vi "PBKDF2.vi"() -> ()   [LabVIEW 2013]
doc: "Implements password-based key derivation functionality, PBKDF2, by using a pseudo-random number generator based on HMACSHA1.\n\nLabVIEW implementation of the C# code example from Microsft's web site @ http://msdn.microsoft.com/en-us/library/system.security.cryptography.rfc2898derivebytes(v=VS.80).aspx\n\n1/17/2011 P. Brooks Originated."
panel:
  out "Decrypted String":string
  in  "MyIterations":i32=1000
  out "encrypted string":string
  in  "Data":string="using System;\nusing System.IO;\nusing System.Text;\nusing System.Security.Cryptography;\n\npublic class rfc2898test\n{\n\t// Generate a key k1 with password pwd1 and salt salt1.\n\t// Generate a key k2 with password pwd1 and salt salt1.\n\t// Encrypt data1 with key k1 using symmetric encryption, creating edata1.\n\t// Decrypt edata1 with key k2 using symmetric decryption, creating data2.\n\t// data2 should equal data1.\n\n\tprivate const string usageText = \"Usage: RFC2898 <password>\\nYou must specify the password for encryption.\\n\";\n\tpublic static void Main(string[] passwordargs)\n\t{\n\t\t//If no file name is specified, write usage text.\n\t\tif (passwordargs.Length == 0)\n\t\t{\n\t\t\tConsole.WriteLine(usageText);\n\t\t}\n\t\telse\n\t\t{\n\t\t\tstring pwd1 = passwordargs[0];\n\t\t\t\n\t\t\tbyte[] salt1 = new byte[] { 0x00, 0x01, 0x02, 0x03, 0x04, 0x05, 0x06, 0xF1, 0xF0, 0xEE, 0x21, 0x22, 0x45};\n\t\t\t//data1 can be a string or contents of a file.\n\t\t\tstring data1 = \"Some test data\";\n\t\t\t//The default iteration count is 1000 so the two methods use the same iteration count.\n\t\t\tint myIterations = 1000;\n\t\t\ttry\n\t\t\t{\n\t\t\t\tRfc2898DeriveBytes k1 = new Rfc2898DeriveBytes(pwd1, salt1,myIterations);\n\t\t\t\tRfc2898DeriveBytes k2 = new Rfc2898DeriveBytes(pwd1, salt1);\n\t\t\t\t// Encrypt the data.\n\t\t\t\tTripleDES encAlg = TripleDES.Create();\n\t\t\t\tencAlg.Key = k1.GetBytes(16);\n\t\t\t\tMemoryStream encryptionStream = new MemoryStream();\n\t\t\t\tCryptoStream encrypt = new CryptoStream(encryptionStream, encAlg.CreateEncryptor(),CryptoStreamMode.Write);\n\t\t\t\tbyte[] utfD1 = new System.Text.UTF8Encoding(false).GetBytes(data1);\n\n\t\t\t\tencrypt.Write(utfD1, 0, utfD1.Length);\n\t\t\t\tencrypt.FlushFinalBlock();\n\t\t\t\tencrypt.Close();\n\t\t\t\tbyte[] edata1 = encryptionStream.ToArray();\n\t\t\t\tk1.Reset();\n\n\t\t\t\t// Try to decrypt, thus showing it can be round-tripped.\n\t\t\t\tTripleDES decAlg = TripleDES.Create();\n\t\t\t\tdecAlg.Key = k2.GetBytes(16);\n\t\t\t\tdecAlg.IV = encAlg.IV;\n\t\t\t\tMemoryStream decryptionStreamBacking = new MemoryStream();\n\t\t\t\tCryptoStream decrypt = new CryptoStream(decryptionStreamBacking,decAlg.CreateDecryptor(), CryptoStreamMode.Write);\n\t\t\t\tdecrypt.Write(edata1, 0, edata1.Length);\n\t\t\t\tdecrypt.Flush();\n\t\t\t\tdecrypt.Close();\n\t\t\t\tk2.Reset();\n\t\t\t\tstring data2 = new UTF8Encoding(false).GetString(decryptionStreamBacking.ToArray());\n\n\t\t\t\tif (!data1.Equals(data2))\n\t\t\t\t{\n\t\t\t\t\tConsole.WriteLine(\"Error: The two values are not equal.\");\n\t\t\t\t}\n\t\t\t\telse\n\t\t\t\t{\n\t\t\t\t\tConsole.WriteLine(\"The two values are equal.\");\n\t\t\t\t\tConsole.WriteLine(\"k1 iterations: {0}\",k1.IterationCount);\n\t\t\t\t\tConsole.WriteLine(\"k2 iterations: {0}\",k2.IterationCount);\n\t\t\t\t}\n\t\t\t}\n\t\t\tcatch (Exception e)\n\t\t\t{\n\t\t\t\tConsole.WriteLine(\"Error: \",e);\n\t\t\t}\n\n\t\t}\n\t}\n}"
  in  "Password":string="PBKDF2"
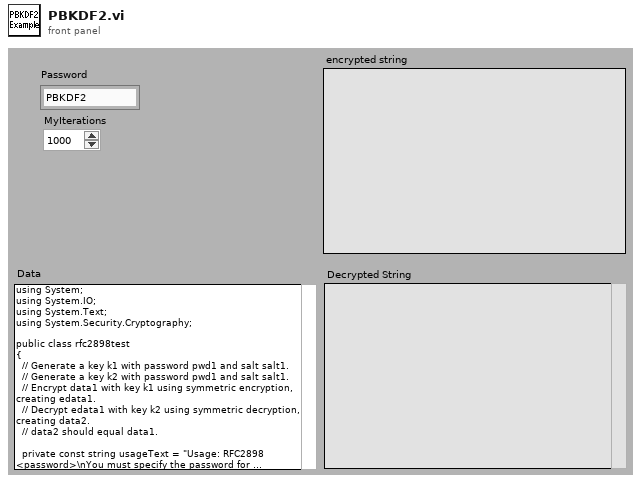
[diagram p1: front panel]
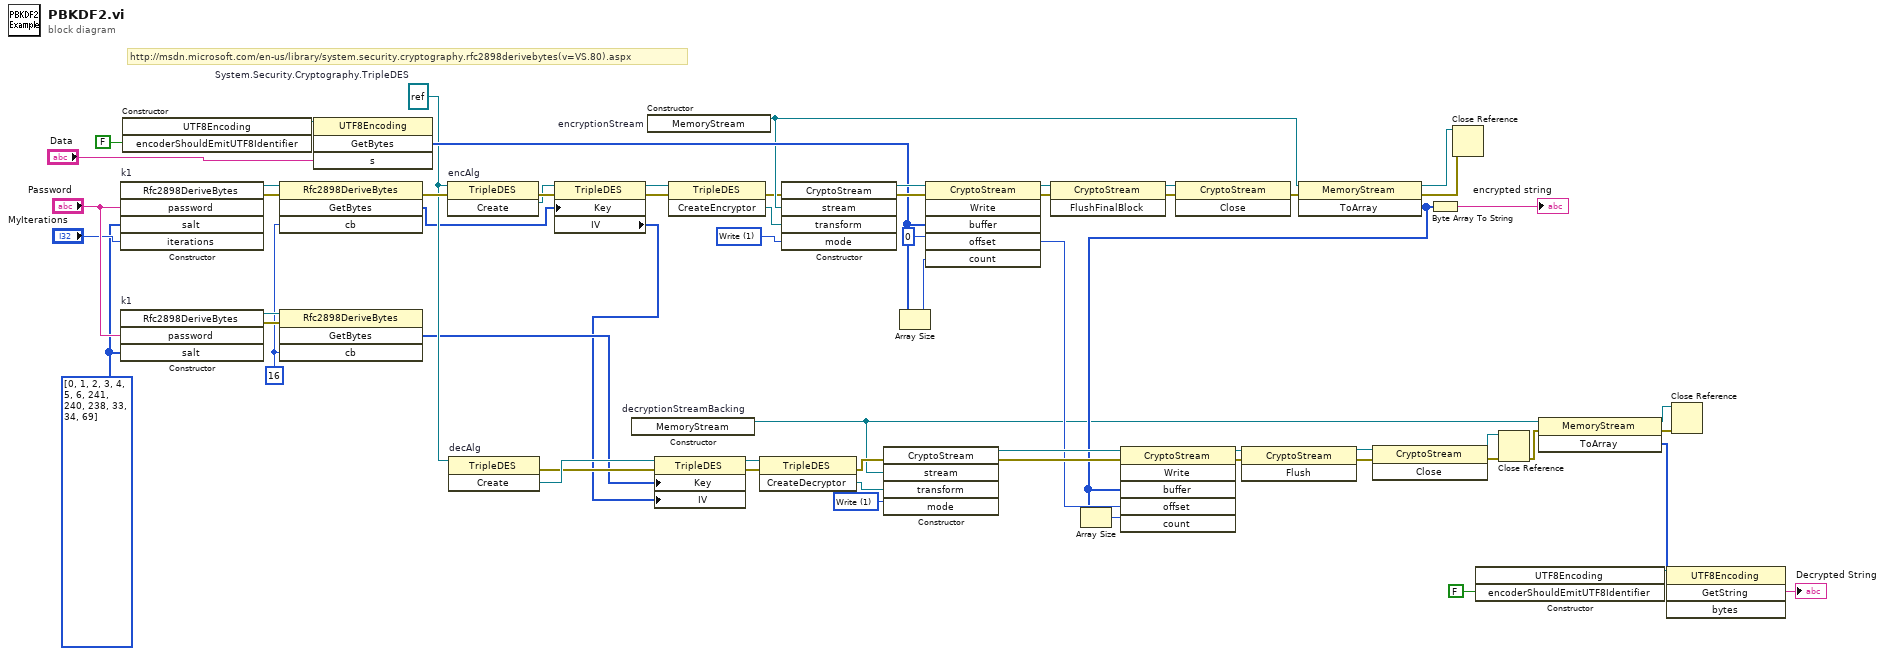
[diagram p0: block diagram]
diagram:
  w30 = 1 items=["Read", "Write"] ("mode")
  w2 = 16 ("cb")
  w27 = 0 ("offset")
  w11 = u8[] [0, 1, 2, 3, 4, 5, 6, 241, 240, 238, 33, 34, 69] ("unsigned byte array")
  w62 = 1 items=["Read", "Write"] ("mode")
  w36 = refnum<k24> refnum  # System.Security.Cryptography.TripleDES
  # "http://msdn.microsoft.com/en-us/library/system.security.cryptography.rfc2898derivebytes(v=VS.80).aspx"
  n1 = constructor on="k1" class="Rfc2898DeriveBytes"("password"="Password", "salt"=w11, "iterations"="MyIterations") -> (reference out=w49:refnum<k24>, error out=w46:errorcluster)  [unwired: 3 in, 4 out]
  n2 = constructor on="k1" class="Rfc2898DeriveBytes"("password"="Password", "salt"=w11) -> (reference out=w39:refnum<k24>, error out=w40:errorcluster)  [unwired: 3 in, 3 out]
  n3 = constructor class="UTF8Encoding"("encoderShouldEmitUTF8Identifier"=FALSE) -> (reference out=w51:refnum<k24>)  [unwired: 3 in, 3 out]
  n4 = invoke class="Rfc2898DeriveBytes" method="GetBytes"(reference=w49, error in=w46, "cb"=w2) -> (error out=w47:errorcluster, "GetBytes"=w16:u8[])  [unwired: 1 in, 2 out]
  n5 = invoke class="Rfc2898DeriveBytes" method="GetBytes"(reference=w39, error in=w40, "cb"=w2) -> ("GetBytes"=w15:u8[])  [unwired: 1 in, 3 out]
  n6 = invoke class="UTF8Encoding" method="GetBytes"(reference=w51, "s"="Data") -> ("GetBytes"=w50:u8[])  [unwired: 2 in, 3 out]
  n7 = invoke on="encAlg" class="TripleDES" method="Create"(reference=w36, error in=w47) -> (error out=w58:errorcluster, "Create"=w57:refnum<k24>)  [unwired: 1 in, 1 out]
  n8 = invoke on="decAlg" class="TripleDES" method="Create"(reference=w36) -> (error out=w37:errorcluster, "Create"=w38:refnum<k24>)  [unwired: 2 in, 1 out]
  n9 = property class="TripleDES"(reference=w57, error in=w58, "Key"=w16) -> (reference out=w56:refnum<k24>, error out=w48:errorcluster, "IV"=w1:u8[])
  n10 = constructor on="decryptionStreamBacking" class="MemoryStream"() -> (reference out=w20:refnum<k24>)  [unwired: 3 in, 2 out]
  n11 = constructor on="encryptionStream" class="MemoryStream"() -> (reference out=w31:refnum<k24>)  [unwired: 3 in, 2 out]
  n12 = property class="TripleDES"(reference=w38, error in=w37, "Key"=w15, "IV"=w1) -> (reference out=w35:refnum<k24>, error out=w34:errorcluster)
  n13 = invoke class="TripleDES" method="CreateEncryptor"(reference=w56, error in=w48) -> (error out=w8:errorcluster, "CreateEncryptor"=w55:refnum<k24>)  [unwired: 1 in, 1 out]
  n14 = invoke class="TripleDES" method="CreateDecryptor"(reference=w35, error in=w34) -> (error out=w33:errorcluster, "CreateDecryptor"=w32:refnum<k24>)  [unwired: 1 in, 1 out]
  n15 = constructor class="CryptoStream"(error in=w8, "stream"=w31, "transform"=w55, "mode"=w62) -> (reference out=w61:refnum<k24>, error out=w59:errorcluster)  [unwired: 2 in, 4 out]
  n16 = constructor class="CryptoStream"(error in=w33, "stream"=w20, "transform"=w32, "mode"=w30) -> (reference out=w29:refnum<k24>, error out=w28:errorcluster)  [unwired: 2 in, 4 out]
  n17 = Array Size(array=w50) -> (size(s)=w60:i32)
  n18 = invoke class="CryptoStream" method="Write"(reference=w61, error in=w59, "buffer"=w50, "offset"=w27, "count"=w60) -> (reference out=w54:refnum<k24>, error out=w45:errorcluster)  [unwired: 1 in, 4 out]
  n19 = invoke class="CryptoStream" method="FlushFinalBlock"(reference=w54, error in=w45) -> (reference out=w43:refnum<k24>, error out=w44:errorcluster)  [unwired: 1 in, 1 out]
  n20 = invoke class="CryptoStream" method="Close"(reference=w43, error in=w44) -> (error out=w42:errorcluster)  [unwired: 1 in, 2 out]
  n21 = invoke class="MemoryStream" method="ToArray"(reference=w31, error in=w42) -> (reference out=w14:refnum<k24>, error out=w13:errorcluster, "ToArray"=w26:u8[])  [unwired: 1 in]
  n22 = Array Size(array=w26) -> (size(s)=w25:i32)
  n23 = invoke class="CryptoStream" method="Write"(reference=w29, error in=w28, "buffer"=w26, "offset"=w27, "count"=w25) -> (reference out=w23:refnum<k24>, error out=w24:errorcluster)  [unwired: 1 in, 4 out]
  n24 = invoke class="CryptoStream" method="Flush"(reference=w23, error in=w24) -> (reference out=w21:refnum<k24>, error out=w22:errorcluster)  [unwired: 1 in, 1 out]
  n25 = invoke class="CryptoStream" method="Close"(reference=w21, error in=w22) -> (reference out=w7:refnum<k24>, error out=w6:errorcluster)  [unwired: 1 in, 1 out]
  n26 = Byte Array To String(unsigned byte array=w26) -> (string=→"encrypted string":string)
  n27 = Close Reference(reference=w14, error in (no error)=w13) -> ()  [unwired: 1 out]
  n28 = constructor class="UTF8Encoding"("encoderShouldEmitUTF8Identifier"=FALSE) -> (reference out=w18:refnum<k24>)  [unwired: 3 in, 3 out]
  n29 = Close Reference(reference=w7, error in (no error)=w6) -> (error out=w5:errorcluster)
  n30 = invoke class="MemoryStream" method="ToArray"(reference=w20, error in=w5) -> (reference out=w4:refnum<k24>, error out=w3:errorcluster, "ToArray"=w10:u8[])  [unwired: 1 in]
  n31 = invoke class="UTF8Encoding" method="GetString"(reference=w18, "bytes"=w10) -> ("GetString"=→"Decrypted String":string)  [unwired: 2 in, 3 out]
  n32 = Close Reference(reference=w4, error in (no error)=w3) -> ()  [unwired: 1 out]
